vi "midiMessageConstant--PitchBend.vi"() -> (2 "Message":u8 format="%.0x")   [LabVIEW 2020, in "midi.lvclass"]
uses:
  midi.lvclass
  midi.lvclass/midi.ctl
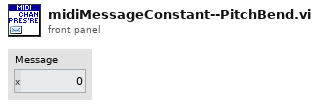
[diagram p1: front panel]
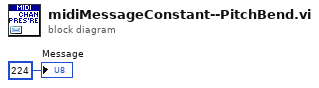
[diagram p0: block diagram]
diagram:
  "Message" <- u8 224 ("Message")
